vi "SetParameterAsChanged.vi"(7 "Qualified Name":string, 8 "error in (no error)":errorcluster, 10 "Keys":string[](array[string]), 11 "ConfigManager in":refnum<class "ConfigManager.lvclass">) -> (0 "error out":errorcluster, 3 "ConfigManager out":refnum<class "ConfigManager.lvclass">)   [LabVIEW 2013, in "CfgManager.lvlib" / "ConfigManager.lvclass"]
uses:
  ConfigManager.lvclass
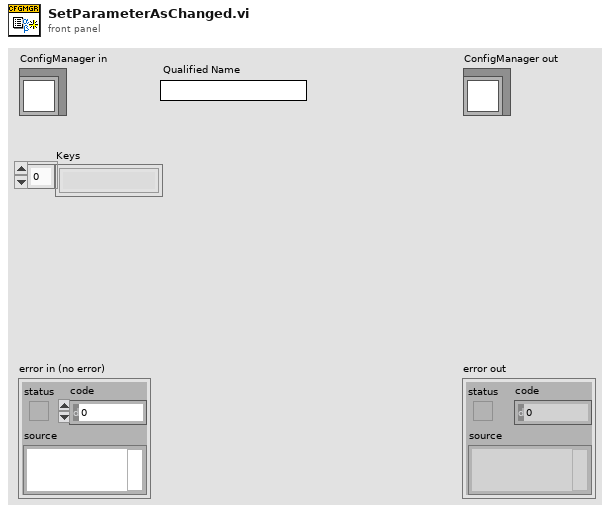
[diagram p1: front panel]
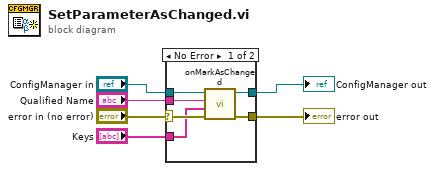
[diagram p0: block diagram]
diagram:
  n1 = case shown="No Error" "error in (no error)" {
    selector: "error in (no error)" -> [w10 w13]
    tunnel: "Qualified Name" -> [w11 _]
    tunnel: "ConfigManager in" -> [w12 w14]
    tunnel: [w7 w14] -> w4
    tunnel: [w8 w13] -> w3
    tunnel: "Keys" -> [w9 _]
    frame No Error {
      n2 = call-dynamic "onMarkAsChanged.vi"("error in (no error)"=w10, "keys"=w9, "Qualified Name"=w11, "ConfigManager in"=w12) -> ("error out"=w8:errorcluster, "ConfigManager out"=w7:refnum<class "ConfigManager.lvclass">)  [unwired: 6 in]
    }
    frame Error {
    }
  }
  "error out" <- w3
  "ConfigManager out" <- w4
